vi "myRIO v1.0 Unreserve DIO.vi"(7 "Allow multiple opens?":bool, 8 "error in (no error)":errorcluster, 10 "DIO Channel List":T2, 11 "myRIO FPGA Ref In":T1) -> (0 "error out":errorcluster)   [LabVIEW 2021]
uses:
  <vilib>/myRIO/Common/Instrument Driver Framework/myRIO v1.0/DIO/typedefs/DIO Channels List.ctl
  <vilib>/myRIO/Common/Instrument Driver Framework/myRIO v1.0/DIO/typedefs/DIO Channels Enum.ctl
  <vilib>/myRIO/Common/Instrument Driver Framework/Utilities/typedefs/Generic FPGA Reference.ctl
  <vilib>/myRIO/Common/Instrument Driver Framework/myRIO v1.0/Resource Manager/vis/myRIO v1.0 Create Configuration List.vi
  <vilib>/myRIO/Common/Instrument Driver Framework/myRIO v1.0/Resource Manager/vis/myRIO v1.0 Unreserve Channel.vi
  <vilib>/myRIO/Common/Instrument Driver Framework/myRIO v1.0/Resource Manager/vis/myRIO v1.0 Build Mutex Name.vi
  <vilib>/myRIO/Common/Instrument Driver Framework/Utilities/vis/Configuration Manager.vi
  <vilib>/myRIO/Common/Instrument Driver Framework/Utilities/vis/IO Manager.vi
  <vilib>/Utility/error.llb/Error Cluster From Error Code.vi
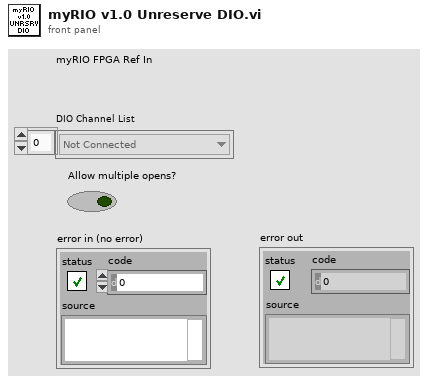
[diagram p1: front panel]
types:
  T1 = typedef "Generic FPGA Reference.ctl" = refnum<k20>
  T2 = typedef "DIO Channels List.ctl" = T3[]
  T3 = typedef "DIO Channels Enum.ctl" = enum16{"Not Connected", "C/DIO0", "C/DIO1", "C/DIO2", "C/DIO3", "C/DIO4", "C/DIO5", "C/DIO6", "C/DIO7", "A/DIO0", "A/DIO1", "A/DIO2", "A/DIO3", "A/DIO4", "A/DIO5", "A/DIO6", "A/DIO7", "A/DIO8", "A/DIO9", "A/DIO10", "A/DIO11", "A/DIO12", "A/DIO13", "A/DIO14", "A/DIO15", "A/DIO16", "A/DIO17", "A/DIO18", "A/DIO19", "B/DIO0", "B/DIO1", "B/DIO2", "B/DIO3", "B/DIO4", "B/DIO5", "B/DIO6", "B/DIO7", "B/DIO8", "B/DIO9", "B/DIO10", "B/DIO11", "B/DIO12", "B/DIO13", "B/DIO14", "B/DIO15", "B/DIO16", "B/DIO17", "B/DIO18", "B/DIO19", "LED0", "LED1", "LED2", "LED3", "Button0", "DIO/DIO0", "DIO/DIO1", "DIO/DIO2", "DIO/DIO3", "DIO/DIO4", "DIO/DIO5", "DIO/DIO6", "DIO/DIO7", "DIO/DIO8", "DIO/DIO9", "SPI/CS0", "SPI/CS1", "SPI/CS2", "SPI/CS3", "LED RADIO (Green)", "LED RADIO (Red)", "LED COMM (Green)", "LED COMM (Red)", "LED MODE (Green)", "LED MODE (Red)"}
  T4 = typedef "myRIO v1.0 Channel Reservation List.ctl" = T5[]
  T5 = typedef "myRIO v1.0 Channel Reservation Info.ctl" = cluster{"Channel Name":string, "Connector":T6, "Mutex ID":i32}
  T6 = typedef "myRIO v1.0 Connector List.ctl" = enum32{"None", "ConnectorA", "ConnectorB", "ConnectorC"}
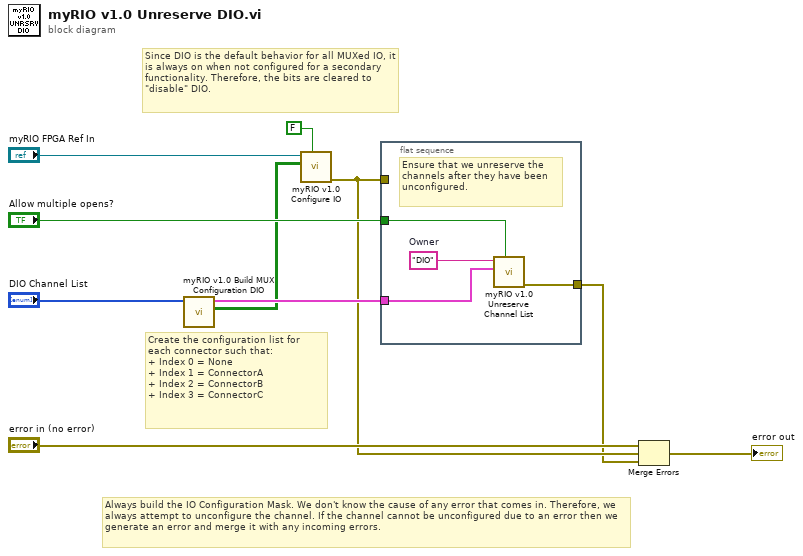
[diagram p0: block diagram]
diagram:
  # "Since DIO is the default behavior for all MUXed IO, it is always on when not configured for a secondary functionality. Therefore, the bits are cleared to \"disable\" DIO."
  # "Always build the IO Configuration Mask. We don't know the cause of any error that comes in. Therefore, we always attempt to unconfigure the channel. If the channel cannot be unconfigured due to an error then we generate an error and merge it with any incoming errors."
  # "Create the configuration list for each connector such that:\n+ Index 0 = None\n+ Index 1 = ConnectorA\n+ Index 2 = ConnectorB \n+ Index 3 = ConnectorC"
  n1 = call <vilib>:"myRIO v1.0 Build MUX Configuration DIO.vi"("DIO Channel List"="DIO Channel List") -> ("Configuration Bitmask Array"=w3:bool[][], "Channel Reservation List"=w4:T4)  [unwired: 9 in]
  n2 = call <vilib>:"myRIO v1.0 Configure IO.vi"("Value"=FALSE ("Clear?"), "Bitmask Array"=w3, "myRIO FPGA Ref In"="myRIO FPGA Ref In") -> ("error out"=w2:errorcluster)  [unwired: 8 in]
  n3 = flat-sequence {
    tunnel: "Allow multiple opens?" -> [w14]
    tunnel: w4 -> [w12]
    tunnel: [w11] -> w1
    tunnel: w2 -> [_]
    frame #0 {
      w13 = "DIO"  # Owner
      # "Ensure that we unreserve the channels after they have been unconfigured."
      n4 = call <vilib>:"myRIO v1.0 Unreserve Channel List.vi"("Allow multiple opens?"=w14, "Channel Reservation List"=w12, "Owner"=w13) -> ("error out"=w11:errorcluster)  [unwired: 8 in]
    }
  }
  n5 = Merge Errors("error in (no error)", w2, w1) -> (→"error out":errorcluster)
